vi "EventLabView.vi"() -> ()   [LabVIEW 2017]
uses:
  <vilib>/Instr/_visa.llb/VISA Configure Serial Port (Instr).vi
panel:
  in  "Start loop while":bool
  in  "delay before read (ms)":u32=500
  in  "Przycisk niepaczek":bool
  out "Response":string
  in  "flow control":u16(ring) items=["None"=0, "XON/XOFF"=1, "RTS/CTS"=2, "DTR/DSR"=4]
  in  "stop bits":u16(ring)=10 items=["1.0"=10, "1.5"=15, "2.0"=20]
  in  "parity":enum16{"None", "Odd", "Even", "Mark", "Space"}(ring)
  in  "data bits":u16=8 min=5 max=8 step=1
  in  "baud rate":u32(ring)=9600 items=["75"=75, "110"=110, "134"=134, "150"=150, "300"=300, "600"=600, "1200"=1200, "1800"=1800, "2400"=2400, "4800"=4800, "7200"=7200, "9600"=9600, "14400"=14400, "19200"=19200, "28800"=28800, "38400"=38400, "56000"=56000, "57600"=57600, "115200"=115200, "128000"=128000, "230400"=230400]
  in  "VISA resource name":refnum<visa-resource-name>="COM1"
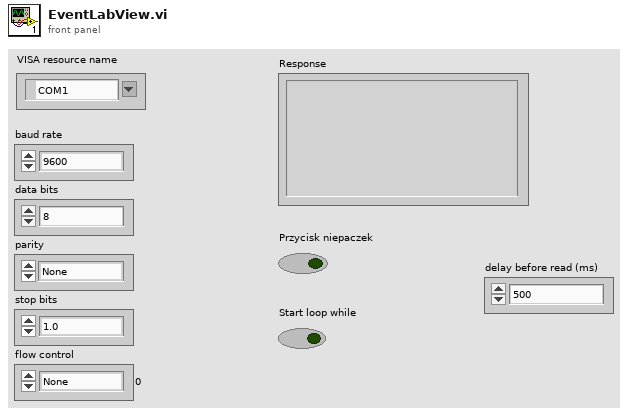
[diagram p1: front panel]
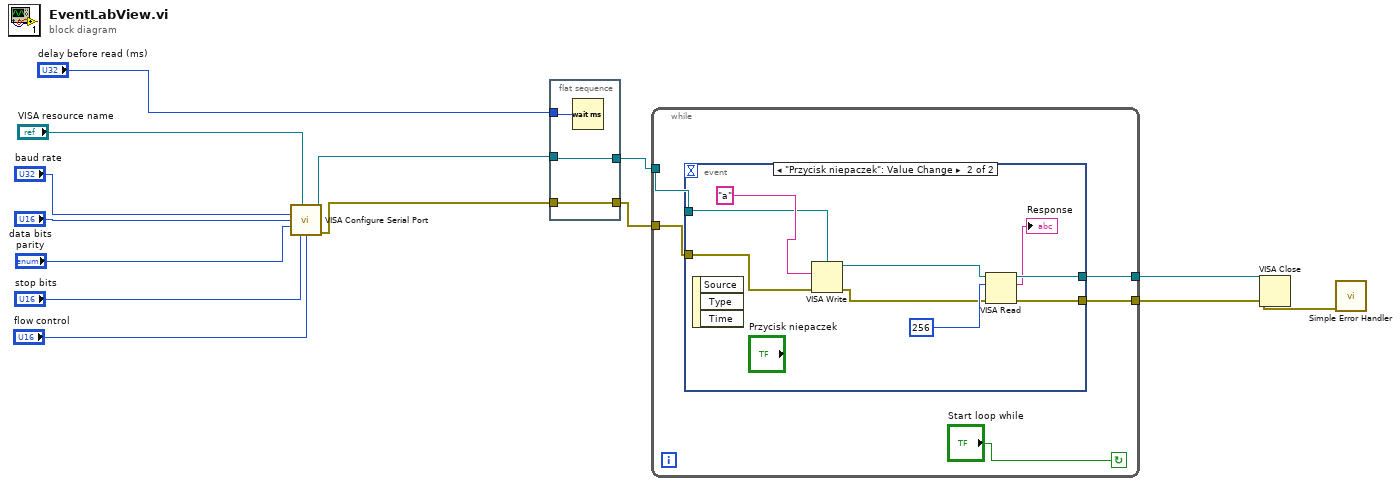
[diagram p0: block diagram]
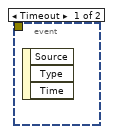
[diagram p2: hidden frame]
diagram:
  n1 = call-poly "VISA Configure Serial Port"("VISA resource name"="VISA resource name", "baud rate (9600)"="baud rate", "data bits (8)"="data bits", "parity (0:none)"="parity", "stop bits (10: 1 bit)"="stop bits", "flow control (0:none)"="flow control") -> ("VISA resource name out"=w5:refnum<visa-resource-name>, "error out"=w6:errorcluster)  [unwired: 3 in, 5 out]
  n2 = flat-sequence {
    tunnel: "delay before read (ms)" -> [w17]
    tunnel: w6 -> [w16]
    tunnel: w5 -> [w15]
    tunnel: [w16] -> w4
    tunnel: [w15] -> w3
    frame #0 {
      n3 = Wait (ms)(milliseconds to wait=w17) -> ()  [unwired: 1 out]
    }
  }
  n4 = while {
    tunnel: w4 -> [w22]
    tunnel: w3 -> [w21]
    tunnel: [w19] -> w2
    tunnel: [w18] -> w1
    stop <- "Start loop while" continue-if-true
    n5 = event shown="[1] \"Przycisk niepaczek\": Value Change" {
      selector: _ -> [_ _]
      dyn-events: _ -> [_ _]
      timeout: _ -> [_ _]
      tunnel: w22 -> [_ w30]
      tunnel: w21 -> [_ w29]
      tunnel: [_ w28] -> w19
      tunnel: [_ w27] -> w18
      event Timeout {
        n6 = event-data() -> ()  [unwired: 1 in, 3 out]
      }
      event "Przycisk niepaczek": Value Change {
        n7 = event-data() -> ()  [unwired: 1 in, 3 out]
        n8 = VISA Write(VISA resource name=w29, write buffer="a", error in (no error)=w30) -> (VISA resource name out=w24:refnum<visa-resource-name>, error out=w25:errorcluster)  [unwired: 1 out]
        n9 = VISA Read(VISA resource name=w24, byte count=256, error in (no error)=w25) -> (VISA resource name out=w27:refnum<visa-resource-name>, read buffer=→"Response":string, error out=w28:errorcluster)  [unwired: 1 out]
      }
    }
  }
  n10 = VISA Close(VISA resource name=w1, error in (no error)=w2) -> (error out=w8:errorcluster)
  n11 = call <vilib>:"Simple Error Handler.vi"("error in (no error)"=w8) -> ()  [unwired: 1 in, 8 out]
